vi "SRV_Build Config File Paths.vi"(0 "Config Dir":path, 5 "Sys Config Name":string) -> (4 "SystemConfig Filepath":path, 6 "MotorsConfig Filepath":path, 8 "SensorsConfig Filepath":path, 12 "SensorsConfig regexp":string, 13 "MotorsConfig regexp":string, 14 "SystemConfig regexp":string)   [LabVIEW 2014]
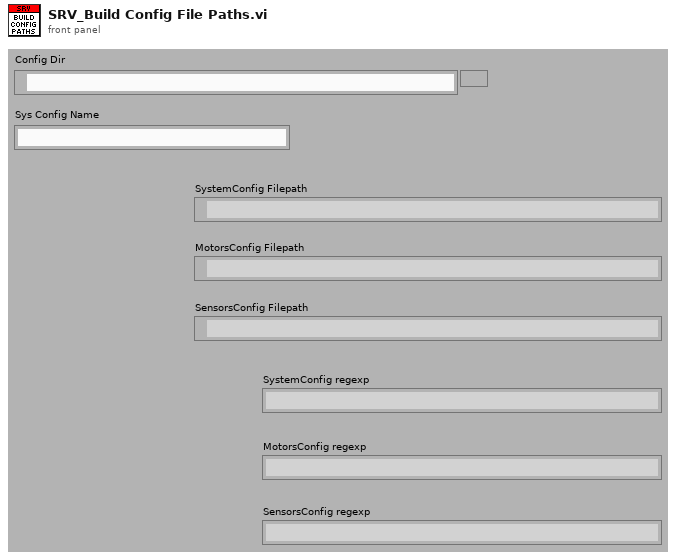
[diagram p1: front panel]
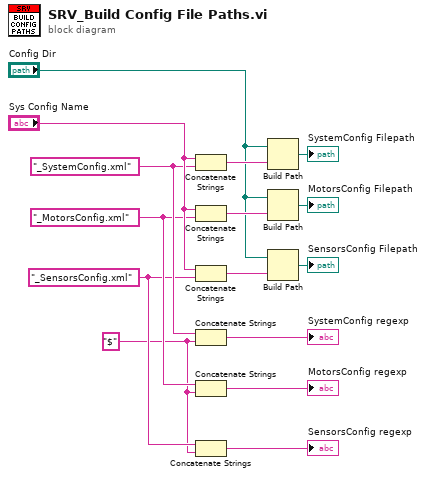
[diagram p0: block diagram]
diagram:
  w1 = "$" ("string")
  w5 = "_SensorsConfig.xml" ("string")
  w6 = "_MotorsConfig.xml" ("string")
  w7 = "_SystemConfig.xml" ("string")
  n1 = Concatenate Strings("Sys Config Name", w7) -> (w14:string)
  n2 = Concatenate Strings("Sys Config Name", w6) -> (w13:string)
  n3 = Concatenate Strings("Sys Config Name", w5) -> (w12:string)
  n4 = Concatenate Strings(w7, w1) -> (→"SystemConfig regexp":string)
  n5 = Concatenate Strings(w6, w1) -> (→"MotorsConfig regexp":string)
  n6 = Concatenate Strings(w5, w1) -> (→"SensorsConfig regexp":string)
  n7 = Build Path(base path="Config Dir", name or relative path=w14) -> (appended path=→"SystemConfig Filepath":path)
  n8 = Build Path(base path="Config Dir", name or relative path=w13) -> (appended path=→"MotorsConfig Filepath":path)
  n9 = Build Path(base path="Config Dir", name or relative path=w12) -> (appended path=→"SensorsConfig Filepath":path)
